vi "Fetch Multi Eval Meas SEM Margin Power Results.vi"(7 "Offset Frequency (Negative)":T1 items=["Negative", "Positive"], 8 "error in (no error)":errorcluster, 9 "Result Type (Current)":i32(ring) items=["Current"=0, "Average"=1, "Minimum"=5], 10 "Instance (1)":T2=1, 11 "VISA resource name":refnum<visa-resource-name>) -> (0 "error out":errorcluster, 1 "SEM Margin Power Results":dbl[](array[numeric]) format="%^.3e", 2 "Reliability":i32, 3 "VISA resource name out":refnum<visa-resource-name>, 4 "Out Of Tolerance":dbl format="%^.3e")   [LabVIEW 2015, in "Rohde&Schwarz CMXP NR FR2 Measurement.lvlib"]
doc: "Returns the spectrum emission trace values at the limit line margin positions of the emission mask areas.\n\nAttributes:\nRSCMXPNRFR2M_ATTR_FETCH_MULTI_EVAL_MEASUREMENT_SEM_NEGATIVE_MARGIN_AVERAGE_POWER_RESULTS\nRSCMXPNRFR2M_ATTR_FETCH_MULTI_EVAL_MEASUREMENT_SEM_POSITIVE_MARGIN_AVERAGE_POWER_RESULTS\nRSCMXPNRFR2M_ATTR_FETCH_MULTI_EVAL_MEASUREMENT_SEM_NEGATIVE_MARGIN_CURRENT_POWER_RESULTS\nRSCMXPNRFR2M_ATTR_FETCH_MULTI_EVAL_MEASUREMENT_SEM_POSITIVE_MARGIN_CURRENT_POWER_RESULTS\nRSCMXPNRFR2M_ATTR_FETCH_MULTI_EVAL_MEASUREMENT_SEM_NEGATIVE_MARGIN_MINIMUM_POWER_RESULTS\nRSCMXPNRFR2M_ATTR_FETCH_MULTI_EVAL_MEASUREMENT_SEM_POSITIVE_MARGIN_MINIMUM_POWER_RESULTS\n\nRemote-control commands:\nFETCh:NRMMw:MEAS<i>:MEValuation:SEMask:MARGin:AVERage:POWer:NEGativ?\nFETCh:NRMMw:MEAS<i>:MEValuation:SEMask:MARGin:AVERage:POWer:POSitiv?\nFETCh:NRMMw:MEAS<i>:MEValuation:SEMask:MARGin:CURRent:POWer:NEGativ?\nFETCh:NRMMw:MEAS<i>:MEValuation:SEMask:MARGin:CURRent:POWer:POSitiv?\nFETCh:NRMMw:MEAS<i>:MEValuation:SEMask:MARGin:MINimum:POWer:NEGativ?\nFETCh:NRMMw:MEAS<i>:MEValuation:SEMask:MARGin:MINimum:POWer:POSitiv?"
uses:
  <instrlib>/Rohde&Schwarz CMXP NR FR2 Measurement/Rohde&Schwarz CMXP NR FR2 Measurement.lvlib
  <instrlib>/Rohde&Schwarz CMXP NR FR2 Measurement/Private/_Instance.ctl
  <instrlib>/Rohde&Schwarz CMXP NR FR2 Measurement/Private/_Offset Frequency.ctl
  <instrlib>/Rohde&Schwarz CMXP NR FR2 Measurement/Private/rsidr_core.llb/rsidr_core.lvlib
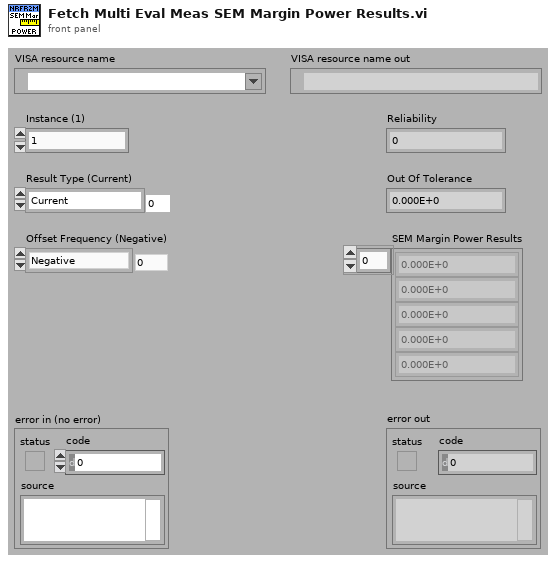
[diagram p1: front panel]
types:
  T1 = typedef "Rohde&Schwarz CMXP NR FR2 Measurement.lvlib/_Offset Frequency.ctl" = i32
  T2 = typedef "Rohde&Schwarz CMXP NR FR2 Measurement.lvlib/_Instance.ctl" = i32
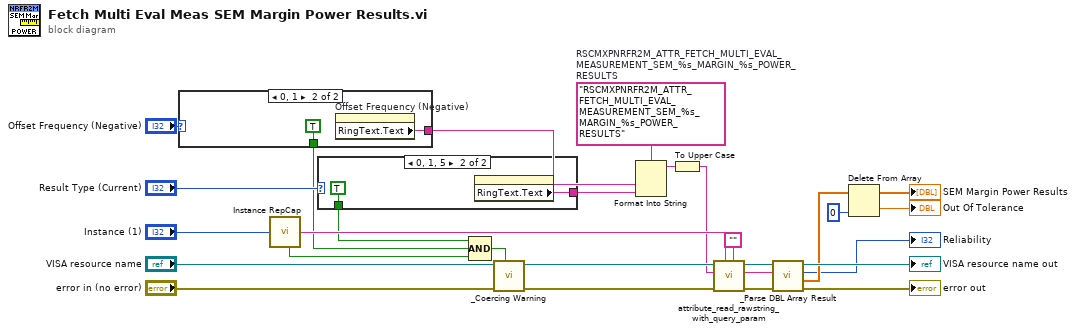
[diagram p0: block diagram]
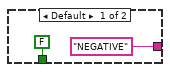
[diagram p2: hidden frame]
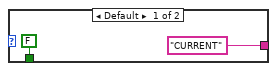
[diagram p3: hidden frame]
diagram:
  w23 = "RSCMXPNRFR2M_ATTR_FETCH_MULTI_EVAL_MEASUREMENT_SEM_%s_MARGIN_%s_POWER_RESULTS"  # RSCMXPNRFR2M_ATTR_FETCH_MULTI_EVAL_MEASUREMENT_SEM_%s_MARGIN_%s_POWER_RESULTS
  n1 = case shown="0, 1" "Offset Frequency (Negative)" {
    tunnel: ["NEGATIVE" w31] -> w4
    tunnel: [FALSE TRUE] -> w3
    frame Default {
    }
    frame 0, 1 {
      n2 = property on="Offset Frequency (Negative)" class="Ring (strict)"() -> ("RingText.Text"=w31:string)  [unwired: 2 in, 2 out]
    }
  }
  n3 = call <instrlib>:"Instance RepCap.vi"("Instance In"="Instance (1)") -> ("In Range?"=w12:bool, "RepCap Identifier Out"=w20:string)  [unwired: 1 in]
  n4 = case shown="0, 1, 5" "Result Type (Current)" {
    tunnel: ["CURRENT" w35] -> w13
    tunnel: [FALSE TRUE] -> w2
    frame Default {
    }
    frame 0, 1, 5 {
      n5 = property on="Result Type (Current)" class="Ring (strict)"() -> ("RingText.Text"=w35:string)  [unwired: 2 in, 2 out]
    }
  }
  n6 = Compound Arithmetic op=AND(w2, w3, w12) -> (w11:bool)
  n7 = call <instrlib>:"_Coercing Warning.vi"("In Range?"=w11, "error in (no error)"="error in (no error)", "VISA resource name"="VISA resource name") -> ("error out"=w22:errorcluster, "VISA resource name out"=w21:refnum<visa-resource-name>)  [unwired: 7 in]
  n8 = Format Into String(format string=w23, w4, w13) -> (resulting string=w19:string)  [unwired: 2 in, 1 out]
  n9 = To Upper Case(1:w19) -> (0:w18:string)
  n10 = call <instrlib>:"attribute_read_rawstring_with_query_param.vi"("Query Parameter (None)"="" ("Empty String Constant"), "Repeated Capability"=w20, "error in"=w22, "Attribute ID"=w18, "VISA resource name"=w21) -> ("error out"=w15:errorcluster, "Raw String out"=w17:string, "VISA resource name out"=w16:refnum<visa-resource-name>)  [unwired: 4 in]
  n11 = call <instrlib>:"_Parse DBL Array Result.vi"("error in (no error)"=w15, "Input String"=w17, "VISA resource name"=w16) -> ("error out"=→"error out":errorcluster, "Results"=w8:dbl[], "Reliability"=→"Reliability":i32, "VISA resource name out"=→"VISA resource name out":refnum<visa-resource-name>)  [unwired: 5 in]
  n12 = Delete From Array(array=w8, index=0) -> (deleted portion=→"Out Of Tolerance":dbl, array with subset deleted=→"SEM Margin Power Results":dbl[])  [unwired: 1 in]
